vi "Magnet_PS_Global.vi"() -> ()   [LabVIEW 2019]
panel:
  out "MagPS_LN2":dbl
  out "MagPS_ST":u32(colorbox)
  out "MagPS_LHe":dbl
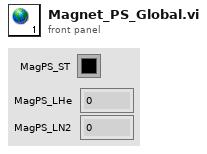
[diagram p1: front panel]
diagram:
